vi "Get Time Only No Spaces.vi"() -> (2 "Time":string)   [LabVIEW 2018]
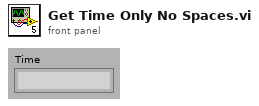
[diagram p1: front panel]
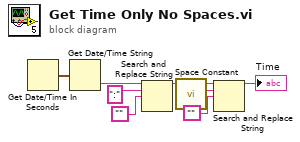
[diagram p0: block diagram]
diagram:
  n1 = Get Date/Time In Seconds() -> (seconds since 1Jan1904=w8:timestamp)
  n2 = Get Date/Time String(seconds (now)=w8) -> (time string=w7:string)  [unwired: 2 in, 1 out]
  n3 = Search and Replace String(input string=w7, search string=":", replace string="") -> (result string=w5:string)  [unwired: 5 in, 3 out]
  n4 = call <vilib>:"Space Constant.vi"() -> ("String"=w2:string)
  n5 = Search and Replace String(input string=w5, search string=w2, replace string="") -> (result string=→"Time":string)  [unwired: 5 in, 3 out]
